vi "mod_Resample (cmplx).vi"(0 "x":cdb[](array[numeric]) format="%.2f", 5 "config":T1={"new sample period"=0.0, "Timing Jitter"=enum."Interpolation", "first point location"=0.0, "prototype filter"={"h"=[], "decimation"=1024.0}} {"prototype filter"."h" format="%.2f"; "prototype filter"."decimation" format="%.2f"; "first point location" format="%.2f"; "new sample period" format="%.2f"}, 13 "Reset? (T)":bool=TRUE) -> (4 "y":cdb[](array[numeric]) format="%.2f", 15 "error out":errorcluster)   [LabVIEW 2020, in "niAMT.lvlib"]
uses:
  <vilib>/addons/Modulation/niAMT.lvlib
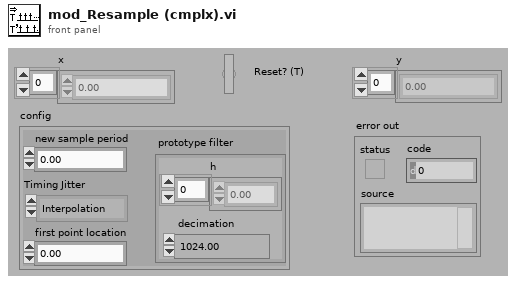
[diagram p1: front panel]
types:
  T1 = cluster{"new sample period":dbl, "Timing Jitter":enum32{"Interpolation", "Rounding"}, "first point location":dbl, "prototype filter":cluster{"h":dbl[], "decimation":dbl}}
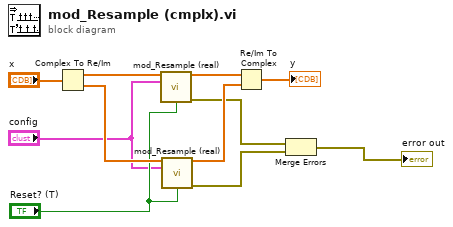
[diagram p0: block diagram]
diagram:
  n1 = Complex To Re/Im(x + iy="x") -> (x=w10:dbl[], y=w9:dbl[])
  n2 = call <vilib>:"mod_Resample (real).vi"("x"=w10, "config"="config", "Reset? (T)"="Reset? (T)") -> ("y"=w7:dbl[], "error out"=w4:errorcluster)  [unwired: 1 in, 10 out]
  n3 = call <vilib>:"mod_Resample (real).vi"("x"=w9, "config"="config", "Reset? (T)"="Reset? (T)") -> ("y"=w6:dbl[], "error out"=w3:errorcluster)  [unwired: 1 in, 10 out]
  n4 = Re/Im To Complex(1:w6, 2:w7) -> (0:→"y":cdb[])
  n5 = Merge Errors(w4, w3) -> (→"error out":errorcluster)
